vi "Main.vi"   [LabVIEW 2016]
uses:
  Source Code/Package ResourceControl/ViHandler/ViHandler.RunModes.ctl
  Source Code/Package ErrorHandling/ErrorHandling.lvclass/ErrorHandling.ctl
  Source Code/Package Libraries/Message Queue/MessageQueue_DequeueElement.vi
  Source Code/Package Libraries/Message Queue/MessageQueue_GetQueue.vi
  Source Code/Package Libraries/Message Queue/MessageQueue_EnqueueElement.vi
  Source Code/Package ErrorHandling/ErrorHandling.checkForErrorAndHandle.vi
  Source Code/Package ErrorHandling/ErrorHandling.GetErrorHandler.vi
  <vilib>/Utility/error.llb/Clear Errors.vi
  Source Code/Package Libraries/StringFunctions/StringFunctions_ReplaceAllBlindSigns.vi
  <vilib>/dlg_ctls.llb/Space Constant.vi
  Source Code/Package Libraries/Message Queue/MessageQueue_ReleaseQueue.vi
  Source Code/Package Libraries/TimingFunctions/TimingFunctions_getUtcTimestamp.vi
  <vilib>/Utility/error.llb/Trim Whitespace.vi
  <vilib>/Utility/error.llb/Search and Replace Pattern.vi
  Source Code/Package ErrorHandling/ErrorHandling.addLastErrorToFile.vi
  Source Code/Package ResourceControl/ViHandler/ViHandler.lvclass
  Source Code/Package ErrorHandling/ErrorHandling.lvclass
  Source Code/Package ResourceControl/ObjectHandler/ObjectHandler.lvclass
  Source Code/Package ResourceControl/CentralStorage/CentralStorage.lvclass
  Source Code/Package Simulation/Modell/Sondenmodell/Sondenmodell.lvclass
  Source Code/Package Simulation/Modell/Hausmodell/Hausmodell.lvclass
  Source Code/Package Simulation/Modell/Umgebung/Umgebung.lvclass
types:
  T1 = typedef "ViHandler.lvclass/ViHandler.RunModes.ctl" = enum16{"FP Closed", "FP Open", "FP Open, Centered"}
  T2 = enum32{"Invalid", "Standard", "Closed", "Hidden", "Minimized", "Maximized"}
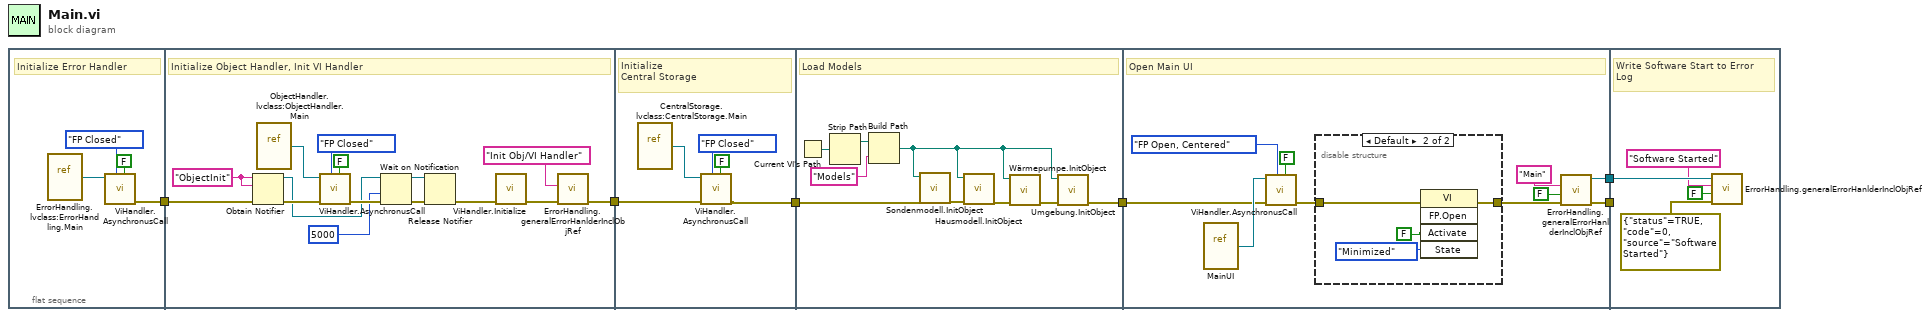
[diagram p0: block diagram]
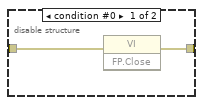
[diagram p2: hidden frame]
diagram:
  n1 = flat-sequence {
    tunnel: [w7] -> w6
    tunnel: w6 -> [w21]
    tunnel: [w13] -> w3
    tunnel: w3 -> [w27]
    tunnel: [w26] -> w2
    tunnel: w2 -> [w35]
    tunnel: [w32] -> w1
    tunnel: [w42] -> w5
    tunnel: [w41] -> w4
    tunnel: w1 -> [w40]
    tunnel: w5 -> [_]
    tunnel: w4 -> [w59]
    frame #0 {
      # "Initialize Error Handler"
      n2 = vi-ref "ErrorHandling.lvclass:ErrorHandling.Main.vi"() -> (w10:refnum<vi>)
      n3 = call "ViHandler.AsynchronusCall.vi"("CheckForExisting?"=FALSE, "Modes"=ViHandler.RunModes."FP Closed", "ViReference"=w10) -> ("error out"=w7:errorcluster)  [unwired: 5 in, 3 out]
    }
    frame #1 {
      w16 = "ObjectInit" ("name (unnamed)")
      # "Initialize Object Handler, Init VI Handler"
      n4 = Obtain Notifier(name (unnamed)=w16, notification data type=w16, error in (no error)=w21) -> (notifier out=w17:refnum<notifier>, error out=w20:errorcluster)  [unwired: 1 in, 1 out]
      n5 = vi-ref "ObjectHandler.lvclass:ObjectHandler.Main.vi"() -> (w25:refnum<vi>)
      n6 = call "ViHandler.AsynchronusCall.vi"("CheckForExisting?"=FALSE, "Modes"=ViHandler.RunModes."FP Closed", "Error In"=w20, "ViReference"=w25) -> ("error out"=w19:errorcluster)  [unwired: 4 in, 3 out]
      n7 = Wait on Notification(notifier=w17, timeout in ms (-1)=5000, error in (no error)=w19) -> (notifier out=w15:refnum<notifier>, error out=w14:errorcluster)  [unwired: 1 in, 2 out]
      n8 = Release Notifier(notifier=w15, error in (no error)=w14) -> (error out=w12:errorcluster)  [unwired: 1 in, 2 out]
      n9 = call "ViHandler.Initialize.vi"("Error In"=w12) -> ("Error out"=w11:errorcluster)  [unwired: 9 in, 1 out]
      n10 = call "ErrorHandling.generalErrorHanlderInclObjRef.vi"("error in"=w11, "Comment(optional)"="Init Obj/VI Handler" ("Comment")) -> ("error out"=w13:errorcluster)  [unwired: 7 in, 2 out]
    }
    frame #2 {
      # "Initialize\nCentral Storage"
      n11 = vi-ref "CentralStorage.lvclass:CentralStorage.Main.vi"() -> (w30:refnum<vi>)
      n12 = call "ViHandler.AsynchronusCall.vi"("CheckForExisting?"=FALSE, "Modes"=ViHandler.RunModes."FP Closed", "Error In"=w27, "ViReference"=w30) -> ("error out"=w26:errorcluster)  [unwired: 4 in, 3 out]
    }
    frame #3 {
      # "Load Models"
      n13 = Current VI's Path() -> (path=w34:path)
      n14 = Strip Path(path=w34) -> (stripped path=w39:path)  [unwired: 1 out]
      n15 = Build Path(base path=w39, name or relative path="Models") -> (appended path=w31:path)
      n16 = call "Sondenmodell.InitObject.vi"("Error In"=w35, "ModelMainPath"=w31) -> ("Error out"=w37:errorcluster)  [unwired: 8 in, 1 out]
      n17 = call "Hausmodell.InitObject.vi"("Error In"=w37, "ModelMainPath"=w31) -> ("Error out"=w36:errorcluster)  [unwired: 8 in, 1 out]
      n18 = call "Wärmepumpe.InitObject.vi"("Error In"=w36, "ModelMainPath"=w31) -> ("Error out"=w33:errorcluster)  [unwired: 8 in, 1 out]
      n19 = call "Umgebung.InitObject.vi"("Error in"=w33, "ModelMainPath"=w31) -> ("Error out"=w32:errorcluster)  [unwired: 8 in, 1 out]
    }
    frame #4 {
      # "Open Main UI"
      n20 = vi-ref "MainUI.vi"() -> (w45:refnum<vi>)
      n21 = call "ViHandler.AsynchronusCall.vi"("CheckForExisting?"=FALSE, "Modes"=ViHandler.RunModes."FP Open, Centered", "Error In"=w40, "ViReference"=w45) -> ("error out"=w43:errorcluster)  [unwired: 4 in, 3 out]
      n22 = disable-structure shown="Default" {
        disable-tunnel: w43 -> [w51 w53]
        disable-tunnel: [w50 w52] -> w49
        frame condition #0 {
          n23 = invoke class="VI" method="FP.Close"(error in=w51) -> (error out=w50:errorcluster)  [unwired: 2 in, 2 out]
        }
        frame condition #1 (active) {
          n24 = invoke class="VI" method="FP.Open"(error in=w53, "Activate"=FALSE ("Activate?"), "State"=T2."Minimized") -> (error out=w52:errorcluster)  [unwired: 2 in, 4 out]
        }
      }
      n25 = call "ErrorHandling.generalErrorHanlderInclObjRef.vi"("error in"=w49, "StopOnError"=FALSE, "Comment(optional)"="Main" ("Comment")) -> ("error out"=w42:errorcluster, "ErrorHandling out"=w41:refnum<data-value>)  [unwired: 6 in, 1 out]
    }
    frame #5 {
      # "Write Software Start to Error Log"
      n26 = call "ErrorHandling.generalErrorHanlderInclObjRef.vi"("error in"=errorcluster {"status"=TRUE, "code"=0, "source"="Software Started"}, "StopOnError"=FALSE, "Comment(optional)"="Software Started" ("Comment"), "ErrorHandling(optional)"=w59) -> ()  [unwired: 5 in, 3 out]
    }
  }
